vi "IsCoordinateConstant.vi"(11 "Coordinate":T1) -> (3 "Constant?":bool)   [LabVIEW 2021]
uses:
  <vilib>/Utility/miscctls.llb/LVPoint32TypeDef.ctl
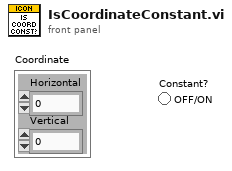
[diagram p1: front panel]
types:
  T1 = typedef "LVPoint32TypeDef.ctl" = cluster{"Horizontal":i32, "Vertical":i32}
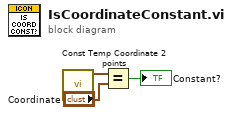
[diagram p0: block diagram]
diagram:
  n1 = call "Const Temp Coordinate 2 points.vi"() -> ("Const Temp Coordinate"=w3:T1)  [unwired: 11 out]
  n2 = Equal?(x=w3, y="Coordinate") -> (x = y?=→"Constant?":bool)
